vi "Read_Dataset(asIn3D_Out1D).vi"(8 "error in":errorcluster, 9 "Validtn Split":sgl=0.1, 10 "Dataset Path(Test)":path, 11 "Dataset Path(Train)":path) -> (0 "error out":errorcluster, 3 "Datasets":T1={"Train"={"Inputs Ref."=variant(refnum<data-value> refnum), "Outputs Ref."=refnum, "Dataset_Size"=0, "Dims_In"={"C"=0, "H"=0, "W"=0}, "Dims_Out"=0, "Labels"=[], "File Paths"=[]}, "Validation"={"Inputs Ref."=variant(refnum<data-value> refnum), "Outputs Ref."=refnum, "Dataset_Size"=0, "Dims_In"={"C"=0, "H"=0, "W"=0}, "Dims_Out"=0, "Labels"=[], "File Paths"=[]}, "Test"={"Inputs Ref."=variant(refnum<data-value> refnum), "Outputs Ref."=refnum, "Dataset_Size"=0, "Dims_In"={"C"=0, "H"=0, "W"=0}, "Dims_Out"=0, "Labels"=[], "File Paths"=[]}})   [LabVIEW 2020]
doc: "Referecens to the dataset (Trainining, Validation and Testing)"
uses:
  <vilib>/Ngene/Deep Learning Toolkit/Toolkit/NN_Data/API/DataSet/DataSet_Types/NN_DataSets_All(In3D_Out1D).ctl
  <vilib>/Ngene/Deep Learning Toolkit/Toolkit/NN_Data/API/DataSet/DataSet_Types/NN_DataSet(In3D_Out1D).ctl
  <vilib>/Ngene/Deep Learning Toolkit/Toolkit/NN_Data/Controls/DataRef_Types/2D/NN_Data_ref(2D_SGL).ctl
  <vilib>/Ngene/Deep Learning Toolkit/Toolkit/NN_Data/API/NN_Dims(C,H,W).ctl
  <vilib>/Analysis/1siggen.llb/Riffle Array (I32).vi
  <vilib>/Ngene/Deep Learning Toolkit/Toolkit/Deep_Learning_Toolkit_by_Ngene.lvlib
  <vilib>/Analysis/NI_AALBase.lvlib
panel:
  # "Instructions:\n1. Download MNISt dataste from http://yann.lecun.com/exdb/mnist/  (4 files with .gz extension)\n2. Exatract all 4 files\n3.  Provide corresponding path to 4 path controls below"
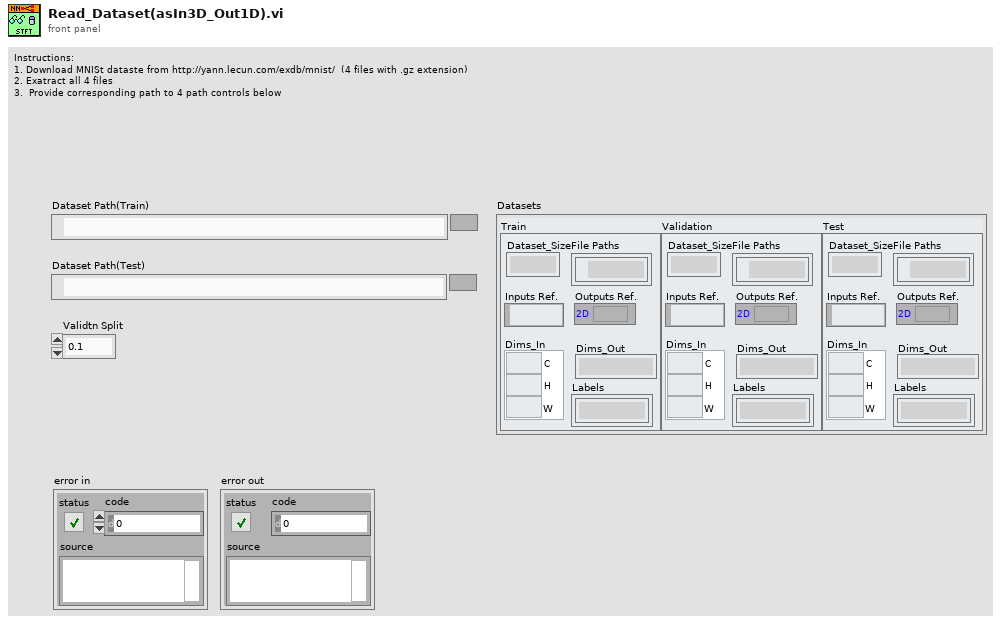
[diagram p1: front panel]
types:
  T1 = typedef "Deep_Learning_Toolkit_by_Ngene.lvlib/NN_DataSets_All(In3D_Out1D).ctl" = cluster{"Train":T2, "Validation":T2, "Test":T2}
  T2 = typedef "Deep_Learning_Toolkit_by_Ngene.lvlib/NN_DataSet(In3D_Out1D).ctl" = cluster{"Inputs Ref.":variant, "Outputs Ref.":T3, "Dataset_Size":i32, "Dims_In":T4, "Dims_Out":i32, "Labels":string[], "File Paths":path[]}
  T3 = typedef "Deep_Learning_Toolkit_by_Ngene.lvlib/NN_Data_ref(2D_SGL).ctl" = refnum<data-value>
  T4 = typedef "Deep_Learning_Toolkit_by_Ngene.lvlib/NN_Dims(C,H,W).ctl" = cluster{"C":i32, "H":i32, "W":i32}
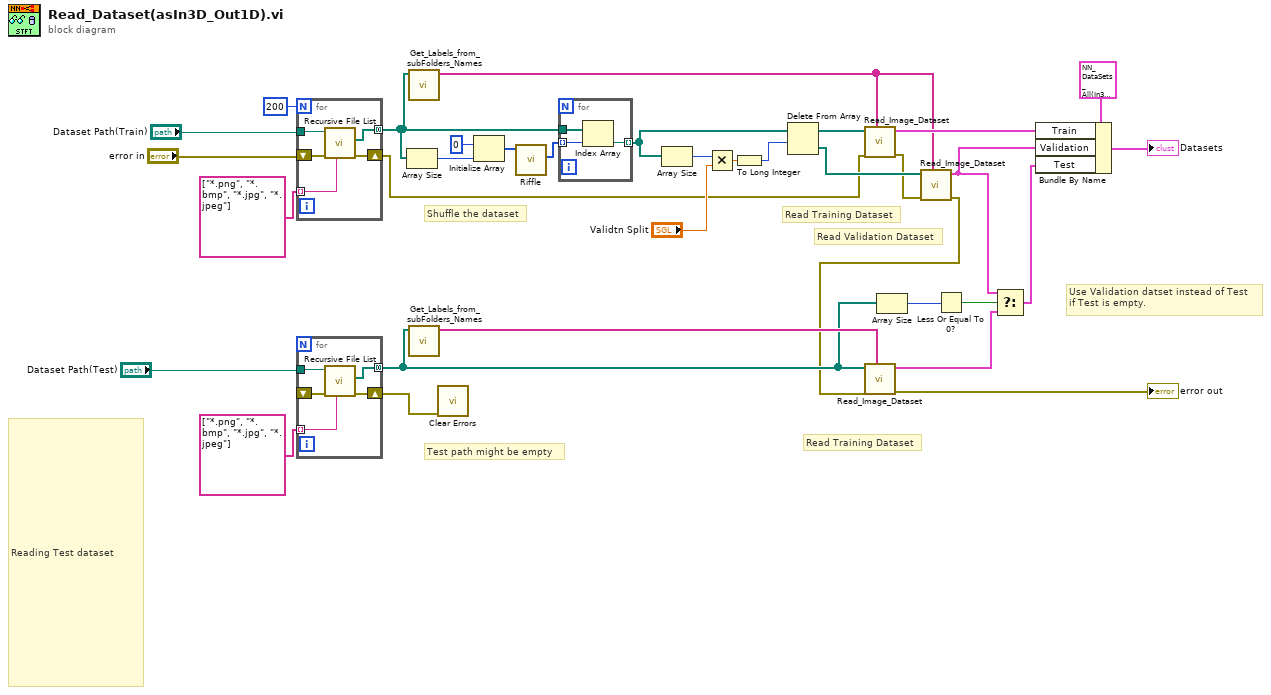
[diagram p0: block diagram]
diagram:
  # "Read Training Dataset"
  # "Test path might be empty"
  # "Read Validation Dataset"
  # "Read Training Dataset"
  # "Shuffle the dataset"
  # "Use Validation datset instead of Test \nif Test is empty."
  # "Reading Test dataset"
  n1 = for {
    N: 200 -> [_]
    tunnel: string[] ["*.png", "*.bmp", "*.jpg", "*.jpeg"] ("pattern") -> [w39] mode=indexing
    tunnel: "Dataset Path(Train)" -> [w37]
    tunnel: [w36] -> w10 mode=concatenating
    shift-right: [w35] -> w15
    shift-left: "error in" -> [w38]
    n2 = call <vilib>:"Recursive File List.vi"("pattern"=w39, "error in (no error)"=w38, "Folder Path"=w37) -> ("error out"=w35:errorcluster, "All Files in Dir"=w36:path[])  [unwired: 4 in, 3 out]
  }
  n3 = for {
    tunnel: string[] ["*.png", "*.bmp", "*.jpg", "*.jpeg"] ("pattern") -> [w44] mode=indexing
    tunnel: "Dataset Path(Test)" -> [w42]
    tunnel: [w41] -> w7 mode=concatenating
    shift-right: [w40] -> w2
    shift-left: _ -> [w43]
    n4 = call <vilib>:"Recursive File List.vi"("pattern"=w44, "error in (no error)"=w43, "Folder Path"=w42) -> ("error out"=w40:errorcluster, "All Files in Dir"=w41:path[])  [unwired: 4 in, 3 out]
  }
  n5 = Array Size(array=w10) -> (size(s)=w23:i32)
  n6 = call "Get_Labels_from_subFolders_Names.vi"("All Files in Dir"=w10) -> ("Labels"=w16:string[])  [unwired: 10 in]
  n7 = call "Get_Labels_from_subFolders_Names.vi"("All Files in Dir"=w7) -> ("Labels"=w11:string[])  [unwired: 10 in]
  n8 = call <vilib>:"Clear Errors.vi"("error in (no error)"=w2) -> ()  [unwired: 5 in, 2 out]
  n9 = Initialize Array(0 ("element"), w23) -> (w27:i32[])
  n10 = call-poly <vilib>:"Riffle.vi"("X"=w27) -> ("Riffled Index"=w26:i32[])  [unwired: 8 in, 2 out]
  n11 = for {
    tunnel: w10 -> [w47]
    tunnel: w26 -> [w46] mode=indexing
    tunnel: [w45] -> w22 mode=indexing
    n12 = Index Array(array=w47, index=w46) -> (element=w45:path)
  }
  n13 = Array Size(array=w22) -> (size(s)=w21:i32)
  n14 = Multiply(x=w21, y="Validtn Split") -> (x*y=w32:sgl)
  n15 = To Long Integer(number=w32) -> (32bit integer=w25:i32)
  n16 = Delete From Array(array=w22, length=w25) -> (deleted portion=w19:path[], array with subset deleted=w20:path[])  [unwired: 1 in]
  n17 = call "Read_Image_Dataset.vi"("Labels"=w16, "error in (no error)"=w15, "Image File Paths"=w20) -> ("error out"=w17:errorcluster, "Dataset Out"=w18:T2)  [unwired: 7 in]
  n18 = Array Size(array=w7) -> (size(s)=w6:i32)
  n19 = call "Read_Image_Dataset.vi"("Labels"=w16, "error in (no error)"=w17, "Image File Paths"=w19) -> ("error out"=w3:errorcluster, "Dataset Out"=w14:T2)  [unwired: 7 in]
  n20 = call "Read_Image_Dataset.vi"("Labels"=w11, "error in (no error)"=w3, "Image File Paths"=w7) -> ("error out"=→"error out":errorcluster, "Dataset Out"=w5:T2)  [unwired: 7 in]
  n21 = Less Or Equal To 0?(x=w6) -> (x <= 0?=w30:bool)
  n22 = Select(t=w14, s=w30, f=w5) -> (s? t:f=w8:T2)
  n23 = Bundle By Name(cluster=T1 {"Train"={"Inputs Ref."=variant(refnum<data-value> refnum), "Outputs Ref."=refnum, "Dataset_Size"=0, "Dims_In"={"C"=0, "H"=0, "W"=0}, "Dims_Out"=0, "Labels"=[], "File Paths"=[]}, "Validation"={"Inputs Ref."=variant(refnum<data-value> refnum), "Outputs Ref."=refnum, "Dataset_Size"=0, "Dims_In"={"C"=0, "H"=0, "W"=0}, "Dims_Out"=0, "Labels"=[], "File Paths"=[]}, "Test"={"Inputs Ref."=variant(refnum<data-value> refnum), "Outputs Ref."=refnum, "Dataset_Size"=0, "Dims_In"={"C"=0, "H"=0, "W"=0}, "Dims_Out"=0, "Labels"=[], "File Paths"=[]}} ("Dataset_Refs_All(In3D_Out1D)"), "Train"=w18, "Validation"=w14, "Test"=w8) -> (→"Datasets":T1)
